vi "LockinRemoteControl.configAO.vi"(8 "error in (no error)":errorcluster, 10 "configAO":T1 {"Channels: AO"."AO f (Hz)" min=0.001 max=10000.0; "Channels: AO"."AO DC (V)" format="%.3p"; "Channels: AO"."AO amp (V)" format="%.3p"}, 11 "RemoteControl":refnum<class "LockinRemoteControl.lvclass">) -> (0 "error out":errorcluster, 3 "RemoteControl out":refnum<class "LockinRemoteControl.lvclass">)   [LabVIEW 2016, in "LockinRemoteControl.lvclass"]
doc: "---------------------------------------------------------------\nJKI State Machine Objects™\nhttp://jki.net/state-machine-objects/\nCopyright (C) 2005-2015, JKI <info@jki.net>\nALL RIGHTS RESERVEDJKI State Machine Objects (SMO) 1.0.0.4\nJKI - JKI\nCopyright (c) 2015, JKI"
uses:
  LockinRemoteControl.lvclass
  Typedefs/PublicEvents--LockinRemoteControl.configAO.ctl
  Instrument.Lockin/Typedefs/AO-cluster.ctl
  Instrument.Lockin/Typedefs/AO_Amp-array.ctl
  Instrument.Lockin/Typedefs/AO_DC-array.ctl
  Instrument.Lockin/Typedefs/AO_f-array.ctl
  Instrument.Lockin/Typedefs/AO_phi-array.ctl
  Instrument.Lockin/Typedefs/Function-array.ctl
  Instrument.Lockin/Typedefs/Function-enum.ctl
  LockinRemoteControl.lvclass/LockinRemoteControl.ctl
  Instrument.Lockin/Instrument.Lockin.lvclass
panel:
  # "For instructions on how to use the JKI State Machine Objects, examples and video tutorials, visit:\nhttp://jki.net/state-machine-objects/\n\nJKI State Machine Objects™\nhttp://jki.net/state-machine-objects/\nCopyright (C) 2005-2015, JKI <info@jki.net>\nALL RIGHTS RESERVED"
  # "1"
  # "2"
  # "3"
  # "4"
  # "5"
  # "6"
  # "7"
  # "8"
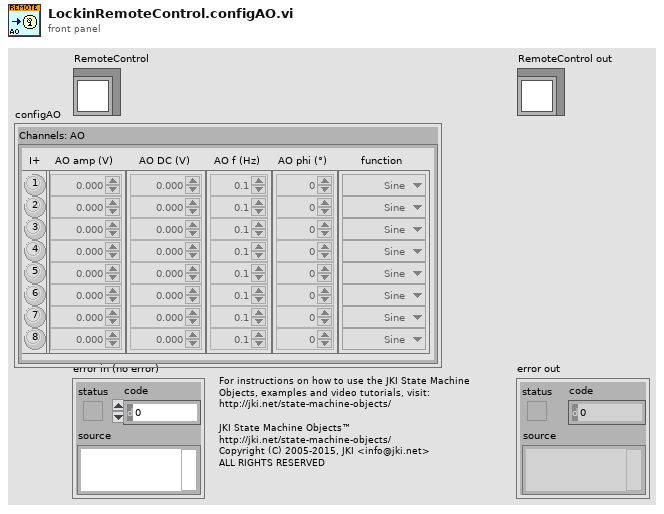
[diagram p1: front panel]
types:
  T1 = typedef "LockinRemoteControl.lvclass/PublicEvents--LockinRemoteControl.configAO.ctl" = cluster{"Channels: AO":T2}
  T2 = typedef "Instrument.Lockin.lvclass/AO-cluster.ctl" = cluster{"AO amp (V)":T3, "AO DC (V)":T4, "AO f (Hz)":T5, "AO phi (°)":T6, "function":T7, "I+":bool[]}
  T3 = typedef "Instrument.Lockin.lvclass/AO_Amp-array.ctl" = dbl[]
  T4 = typedef "Instrument.Lockin.lvclass/AO_DC-array.ctl" = dbl[]
  T5 = typedef "Instrument.Lockin.lvclass/AO_f-array.ctl" = dbl[]
  T6 = typedef "Instrument.Lockin.lvclass/AO_phi-array.ctl" = dbl[]
  T7 = typedef "Instrument.Lockin.lvclass/Function-array.ctl" = T8[]
  T8 = typedef "Instrument.Lockin.lvclass/Function-enum.ctl" = enum16{"Sine", "Triangle", "Square", "Sawtooth"}
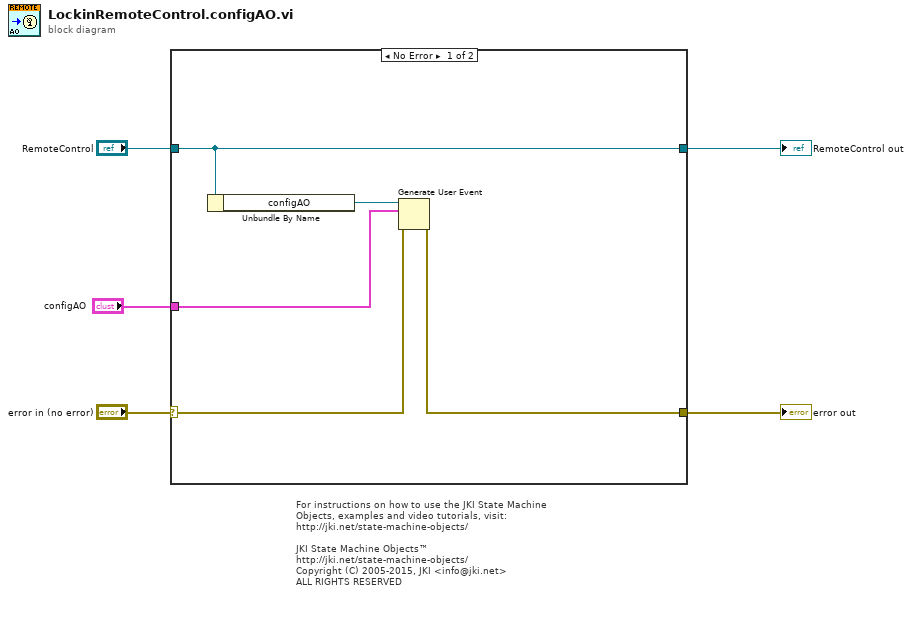
[diagram p0: block diagram]
diagram:
  # "For instructions on how to use the JKI State Machine Objects, examples and video tutorials, visit:\nhttp://jki.net/state-machine-objects/\n\nJKI State Machine Objects™\nhttp://jki.net/state-machine-objects/\nCopyright (C) 2005-2015, JKI <info@jki.net>\nALL RIGHTS RESERVED"
  n1 = case shown="No Error" "error in (no error)" {
    selector: "error in (no error)" -> [w10 w12]
    tunnel: [w7 w12] -> w4
    tunnel: [w6 w11] -> w5
    tunnel: "RemoteControl" -> [w6 w11]
    tunnel: "configAO" -> [w9 _]
    frame No Error {
      n2 = Unbundle By Name(w6) -> ("configAO"=w8:refnum<user-event>)
      n3 = Generate User Event(user event=w8, event data cluster=w9, error in=w10) -> (error out=w7:errorcluster)  [unwired: 1 in, 1 out]
    }
    frame Error {
    }
  }
  "error out" <- w4
  "RemoteControl out" <- w5
